vi "Send TCP Cmd.vi"(8 "error in (no error)":errorcluster, 10 "tcp ref":refnum<k5>, 11 "Queue in":refnum<queue>) -> (0 "error out":errorcluster)   [LabVIEW 2016, in "Vision Server.lvclass"]
uses:
  Vision Server.lvclass
  typedef/Message Type.ctl
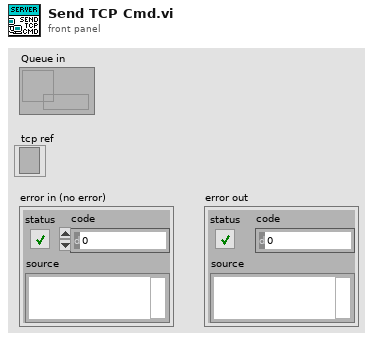
[diagram p1: front panel]
types:
  T1 = typedef "Vision Server.lvclass/Message Type.ctl" = cluster{"type":string, "message":string}
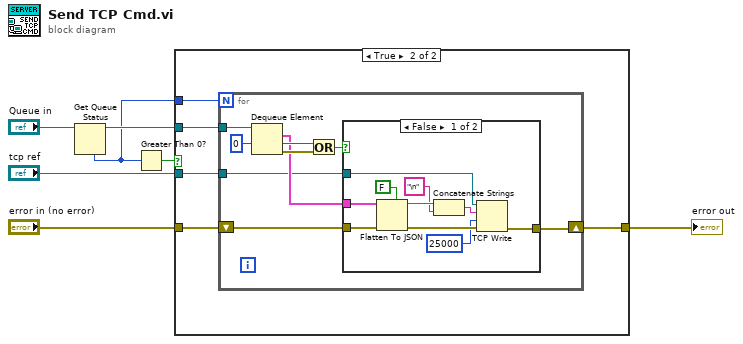
[diagram p0: block diagram]
diagram:
  n1 = Get Queue Status(queue="Queue in") -> (queue out=w3:refnum<queue>, # elements in queue=w1:i32)  [unwired: 2 in, 6 out]
  n2 = Greater Than 0?(x=w1) -> (x > 0?=w2:bool)
  n3 = case shown="True" w2 {
    tunnel: "tcp ref" -> [_ w13]
    tunnel: [w8 w12] -> w6
    tunnel: "error in (no error)" -> [w8 w11]
    tunnel: w3 -> [_ w10]
    tunnel: w1 -> [_ w9]
    frame False {
    }
    frame True {
      n4 = for {
        N: w9 -> [_]
        tunnel: w10 -> [w20]
        shift-right: [w18] -> w12
        shift-left: w11 -> [w16]
        tunnel: w13 -> [w15]
        n5 = Dequeue Element(queue=w20, timeout in ms (-1)=0) -> (element=w17:T1, timed out?=w22:bool, error out=w21:errorcluster)  [unwired: 1 in, 1 out]
        n6 = Or(x=w22, y=w21) -> (x .or. y?=w14:bool)
        n7 = case shown="False" w14 {
          tunnel: [w32 w33] -> w18
          tunnel: w17 -> [w31 _]
          tunnel: w16 -> [w30 w33]
          tunnel: w15 -> [w28 _]
          frame False {
            n8 = Flatten To JSON(enable LabVIEW extensions? (T)=FALSE, anything=w31, error in (no error)=w30) -> (JSON string=w26:string, 11:w29:errorcluster)
            n9 = Concatenate Strings(w26, "\n" ("string")) -> (w25:string)
            n10 = TCP Write(connection ID=w28, data in=w25, error in (no error)=w29, 9:25000 ("timeout ms (25000)")) -> (error out=w32:errorcluster)  [unwired: 2 out]
          }
          frame True {
          }
        }
      }
    }
  }
  "error out" <- w6
